vi "GetAllFiles.vi"(11 "Source Directory":path=path "Z:/work/git/ScreenShotGen") -> (2 "Sub-Directories":path[](array[path]), 3 "Files":path[](array[path]))   [LabVIEW 2017]
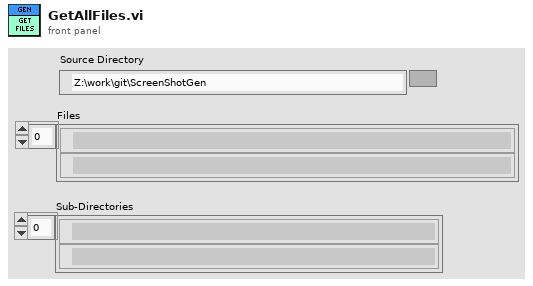
[diagram p1: front panel]
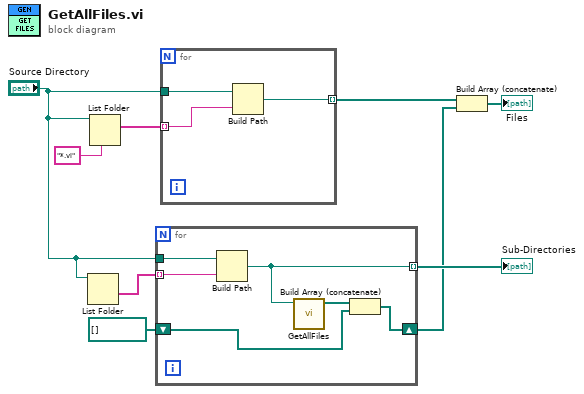
[diagram p0: block diagram]
diagram:
  n1 = List Folder(path="Source Directory") -> (folder names=w2:string[])  [unwired: 3 in, 3 out]
  n2 = List Folder(path="Source Directory", pattern="*.vi") -> (filenames=w9:string[])  [unwired: 2 in, 3 out]
  n3 = for {
    tunnel: w2 -> [w15] mode=indexing
    tunnel: [w14] -> w7 mode=indexing
    shift-right: [w12] -> w4
    shift-left: path[] [] -> [w11]
    tunnel: "Source Directory" -> [w10]
    n4 = Build Path(base path=w10, name or relative path=w15) -> (appended path=w14:path)
    n5 = call "GetAllFiles.vi"("Source Directory"=w14) -> ("Files"=w13:path[])  [unwired: 9 in, 1 out]
    n6 = Build Array (concatenate)(w13, w11) -> (w12:path[])
  }
  "Sub-Directories" <- w7
  n7 = for {
    tunnel: w9 -> [w18] mode=indexing
    tunnel: "Source Directory" -> [w17]
    tunnel: [w16] -> w6 mode=indexing
    n8 = Build Path(base path=w17, name or relative path=w18) -> (appended path=w16:path)
  }
  n9 = Build Array (concatenate)(w6, w4) -> (→"Files":path[])
